vi "main.vi"() -> ()   [LabVIEW 2016]
uses:
  System Status.ctl
  Position Control.ctl
  Position Coordinate.ctl
  Manual Operation Control.ctl
panel:
  in  "Manual Operation Control":T1 {"Speed Override (%)" min=0.0 max=150.0 step=1.0 scale=0.0..150.0; "Rotative"."Step Length" min=0.01 max=100.0 step=0.01; "Rotative"."Speed" scale=0.0..500.0; "Linear"."Step Length" min=0.01 max=500.0 step=0.01; "Linear"."Speed" scale=0.0..500.0}
  in  "Settings":bool
  in  "Stop":bool
  in  "Initialize":bool
  in  "Auto Run":bool
  in  "Auto Run Control":T2[](array[typedef])
  in  "Rev Position":T3={"Pos X"=0.0, "Position Name"="Rel Move", "Pos Y"=0.0, "Pos Z"=0.0, "Pos A"=0.0, "OK Button"=FALSE, "Normal Move"=FALSE, "Fast Move"=FALSE} {"Pos A" format="%.2f"; "Pos Z" format="%.2f"; "Pos Y" format="%.2f"; "Pos X" format="%.2f"}
  in  "Abs Position":T3={"Pos X"=0.0, "Position Name"="Abs Move", "Pos Y"=0.0, "Pos Z"=0.0, "Pos A"=0.0, "OK Button"=FALSE, "Normal Move"=FALSE, "Fast Move"=FALSE} {"Pos A" format="%.2f"; "Pos Z" format="%.2f"; "Pos Y" format="%.2f"; "Pos X" format="%.2f"}
  out "System Status":T4 {"Axis A"."Position" format="%.2g"; "Axis Z"."Position" format="%.2g"; "Axis Y"."Position" format="%.2g"; "Linear Speed" format="%#.2g"; "Axis X"."Position" format="%.2g"}
  out "Error Information":string
  in  "MotionLibrary Path":path=path "C:/Program Files (x86)/National Instruments/LabVIEW 2016/user.lib/iselmotion/CNCAPI/CtrlDll/Dummy/mctlDummy.dll"
  out "Motor hModule":i32
  in  "MotionIni File In":path=path "C:/Program Files (x86)/National Instruments/LabVIEW 2016/user.lib/iselmotion/CNCAPI/CtrlDll/Dummy/MctlDummy.INI"
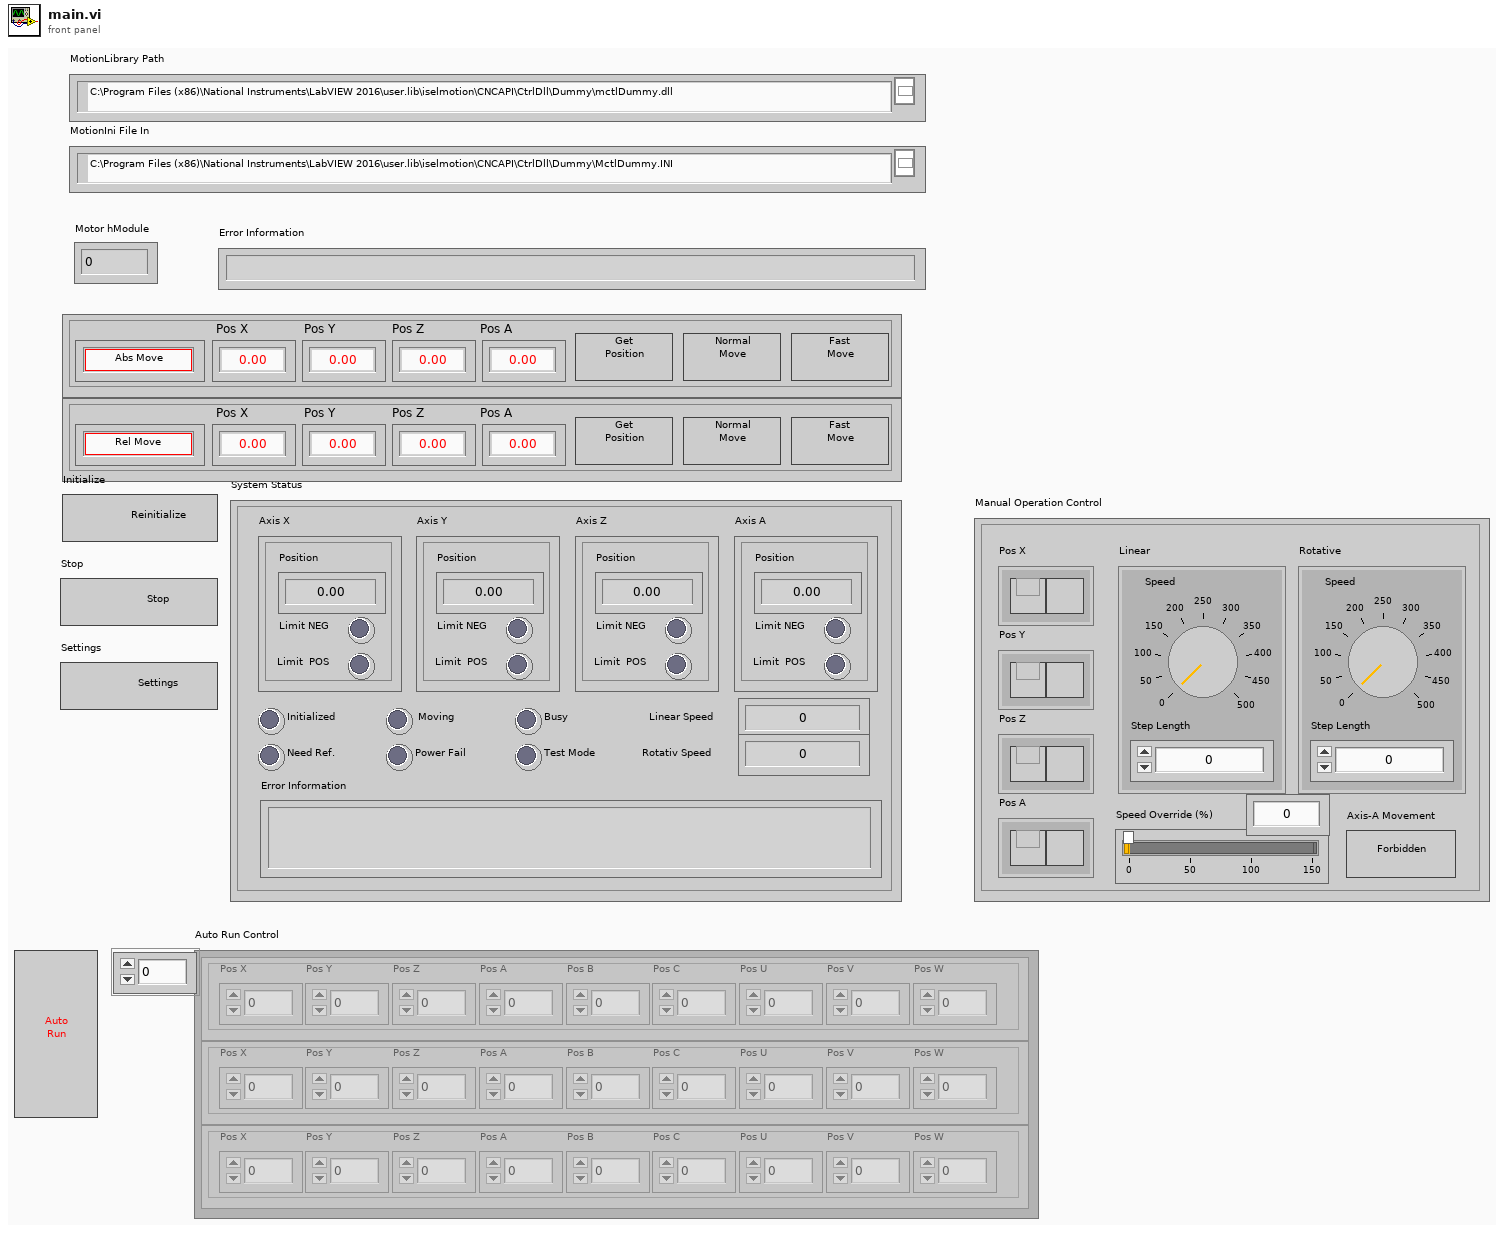
[diagram p1: front panel]
types:
  T1 = typedef "Manual Operation Control.ctl" = cluster{"Pos X":cluster{"Plus":bool, "Minus":bool}, "Pos Y":cluster{"Plus":bool, "Minus":bool}, "Pos Z":cluster{"Plus":bool, "Minus":bool}, "Pos A":cluster{"Plus":bool, "Minus":bool}, "Linear":cluster{"Speed":dbl, "Step Length":dbl}, "Rotative":cluster{"Speed":dbl, "Step Length":dbl}, "Speed Override (%)":dbl, "Axis-A Movement":bool}
  T2 = typedef "Position Coordinate.ctl" = cluster{"Pos X":dbl, "Pos Y":dbl, "Pos Z":dbl, "Pos A":dbl, "Pos B":dbl, "Pos C":dbl, "Pos U":dbl, "Pos V":dbl, "Pos W":dbl}
  T3 = typedef "Position Control.ctl" = cluster{"Pos X":dbl, "Position Name":string, "Pos Y":dbl, "Pos Z":dbl, "Pos A":dbl, "OK Button":bool, "Normal Move":bool, "Fast Move":bool}
  T4 = typedef "System Status.ctl" = cluster{"Axis X":cluster{"Position":dbl, "Limit NEG":bool, "Limit  POS":bool}, "Axis Y":cluster{"Position":dbl, "Limit NEG":bool, "Limit  POS":bool}, "Axis Z":cluster{"Position":dbl, "Limit NEG":bool, "Limit  POS":bool}, "Axis A":cluster{"Position":dbl, "Limit NEG":bool, "Limit  POS":bool}, "Initialized":bool, " Moving":bool, "Busy":bool, "Need Ref.":bool, "Power Fail":bool, "Test Mode":bool, "Linear Speed":dbl, "Rotativ Speed":dbl, "Error Information":string}
  T5 = enum16{"open", "replace", "create", "open or create", "replace or create", "replace or create with confirmation"}
  T6 = cluster{"PosX":i32, "PosY":i32, "PosZ":i32, "PosA":i32, "PosB":i32, "PosC":i32, "PosU":i32, "PosV":i32, "PosW":i32}
  T7 = cluster{"MotionLibrary Path":path, "MotionIni File In":path}
  T8 = cluster{"Common":cluster{"INMOTION":bool, "INSTOPMODE":bool, "INTEACHMODE":bool, "INTESTMODE":bool, "CURRENTOFF":bool, "INPATHMOTION":bool, "ISMOVING":bool, "PATHSTARTED":bool, "NEEDREFERENCERUN":bool, "BREAKERROR":bool, "HWLSACTIVE":bool, "SWLSACTIVE":bool, "HWLSDURINGMOTION":bool, "AFTERRUNERROR":bool, "LOADPATHDATAERROR":bool, "KEYSWITCHERROR":bool, "KEYSWDURINGMOTION":bool, "POWER_FAIL":bool, "SC_FAIL":bool, "HARDWARE_FAIL":bool, "COMMUNICATION_FAIL":bool}, "HWLSNeg":cluster{"HWLS_X_NEG":bool, "HWLS_Y_NEG":bool, "HWLS_Z_NEG":bool, "HWLS_A_NEG":bool, "HWLS_B_NEG":bool, "HWLS_C_NEG":bool, "HWLS_U_NEG":bool, "HWLS_V_NEG":bool, "HWLS_W_NEG":bool}, "HWLSPos":cluster{"HWLS_X_POS":bool, "HWLS_Y_POS":bool, "HWLS_Z_POS":bool, "HWLS_A_POS":bool, "HWLS_B_POS":bool, "HWLS_C_POS":bool, "HWLS_U_POS":bool, "HWLS_V_POS":bool, "HWLS_W_POS":bool}, "SWLSNeg":cluster{"SWLS_X_NEG":bool, "SWLS_Y_NEG":bool, "SWLS_Z_NEG":bool, "SWLS_A_NEG":bool, "SWLS_B_NEG":bool, "SWLS_C_NEG":bool, "SWLS_U_NEG":bool, "SWLS_V_NEG":bool, "SWLS_W_NEG":bool}, "SWLSPos":cluster{"SWLS_X_POS":bool, "SWLS_Y_POS":bool, "SWLS_Z_POS":bool, "SWLS_A_POS":bool, "SWLS_B_POS":bool, "SWLS_C_POS":bool, "SWLS_U_POS":bool, "SWLS_V_POS":bool, "SWLS_W_POS":bool}, "Extended":cluster{"ISBUSY":bool, "DISABLED":bool, "ISINITIALIZED":bool, "READY":bool, "DRILLCYCLEACTIVE":bool, "CTRLSPECERROR":bool}, "Additional flags":cluster{"InMotion":bool, "InStopMode":bool, "InTeachMode":bool, "InTestMode":bool, "CurrentOff":bool, "InPathMotion":bool, "IsMoving":bool, "NeedReferenceRun":bool, "BreakError":bool, "HWLSActive":bool, "SWLSActive":bool, "HWLSDuringMotion":bool, "AfterRunError":bool, "PowerFail":bool, "SCFail":bool, "IsBusy":bool, "Initialized":bool, "Disabled":bool, "HardwareFail":bool, "CommunicationFail":bool, "DrillCycleActive":bool, "CtrlSpecError":bool, "PathStarted":bool}}
  T9 = cluster{"PosX":dbl, "PosY":dbl, "PosZ":dbl, "PosA":dbl, "PosB":dbl, "PosC":dbl, "PosU":dbl, "PosV":dbl, "PosW":dbl}
  T10 = cluster{"PosX":dbl, "HWLS_X_NEG":bool, "HWLS_X_POS":bool}
  T11 = cluster{"PosY":dbl, "HWLS_Y_NEG":bool, "HWLS_Y_POS":bool}
  T12 = cluster{"PosZ":dbl, "HWLS_Z_NEG":bool, "HWLS_Z_POS":bool}
  T13 = cluster{dbl, "HWLS_A_NEG":bool, "HWLS_A_POS":bool}
  T14 = cluster{"LiNormVel":i32, "DrNormVel":i32, "LiFastVel":i32, "DrFastVel":i32, "LiTeachVel":i32, "DrTeachVel":i32, "LiActVel":i32, "DrActVel":i32}
  T15 = cluster{"LiNormVel":dbl, "DrNormVel":dbl, "LiFastVel":dbl, "DrFastVel":dbl, "LiTeachVel":dbl, "DrTeachVel":dbl, "LiActVel":dbl, "DrActVel":dbl}
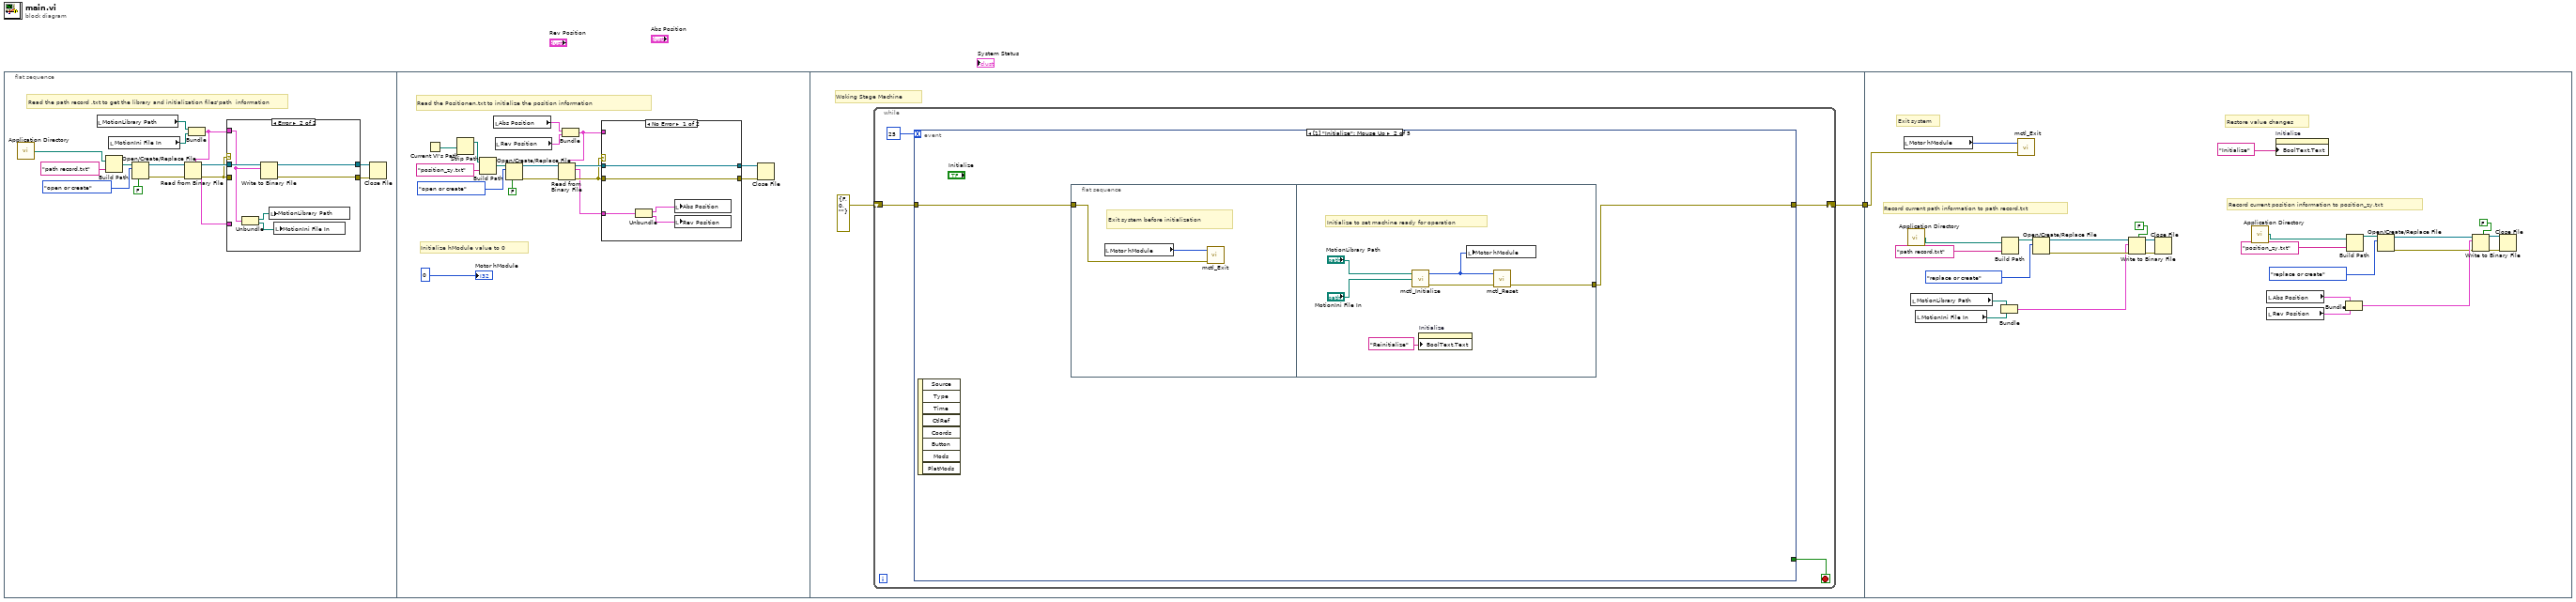
[diagram p0: block diagram]
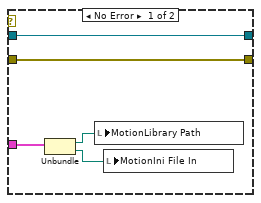
[diagram p2: hidden frame]
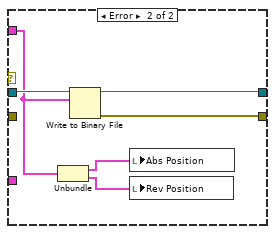
[diagram p3: hidden frame]
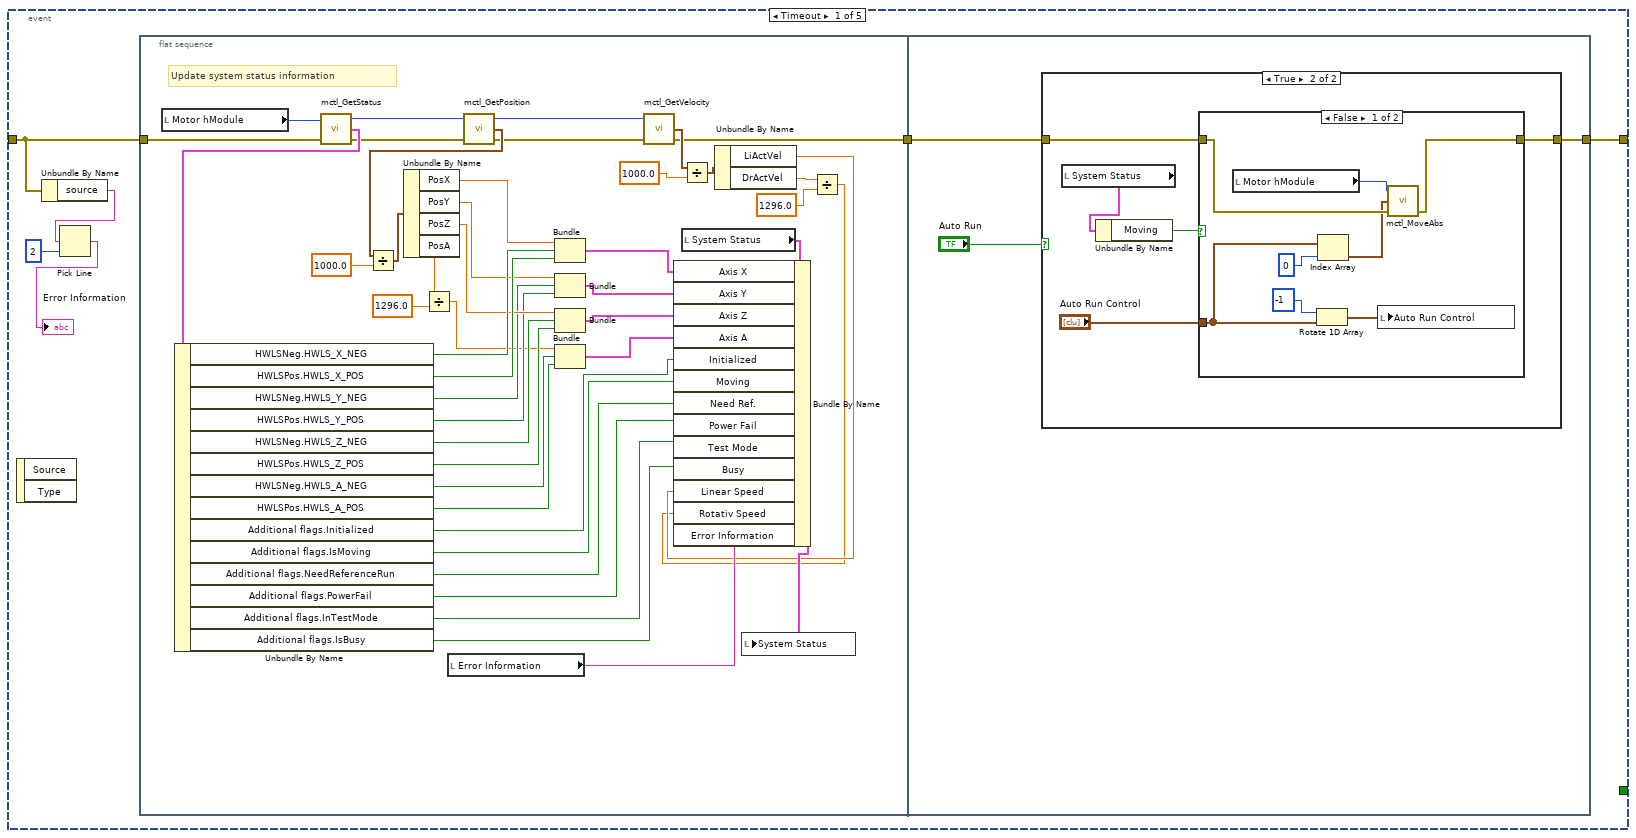
[diagram p4: hidden frame]
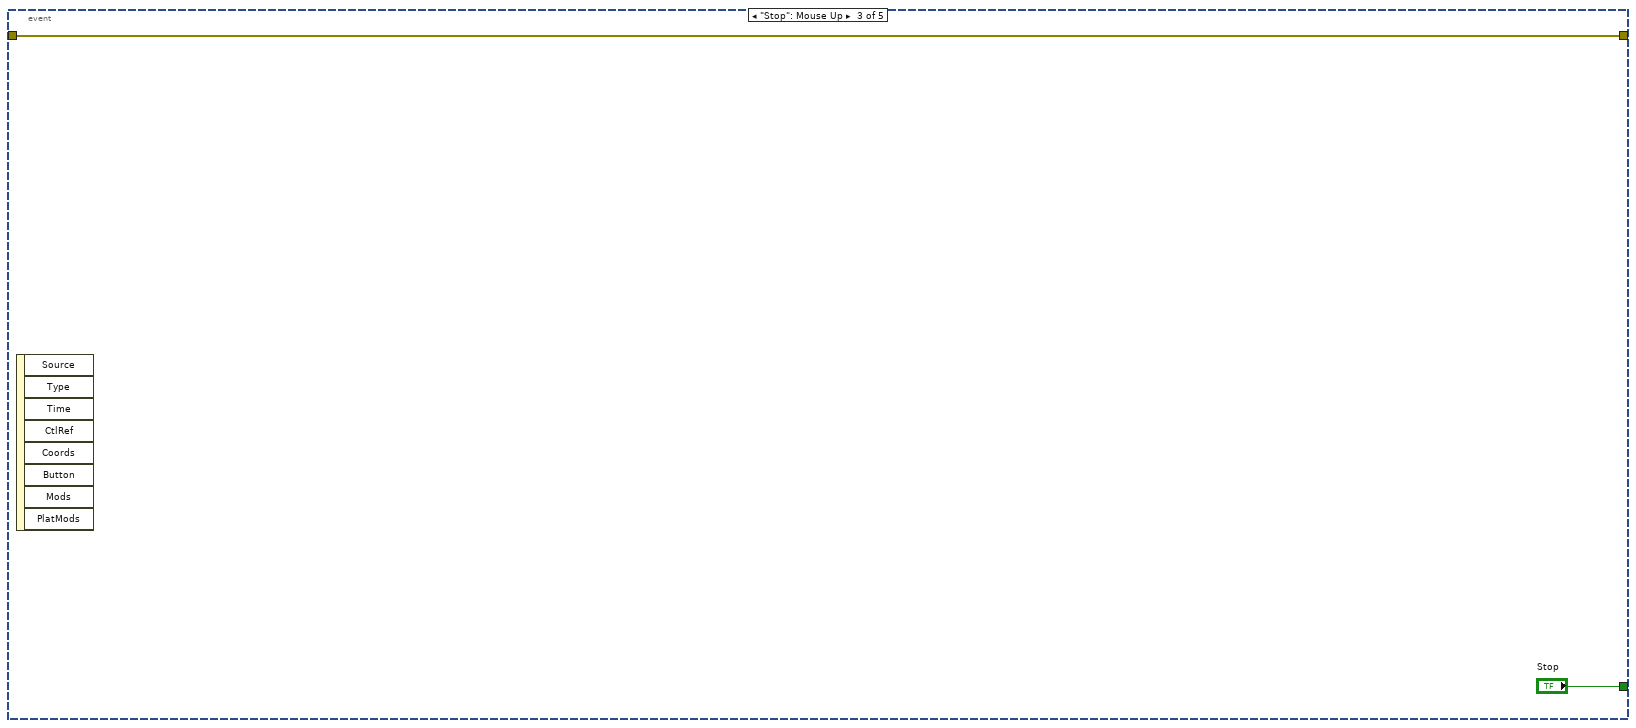
[diagram p7: hidden frame]
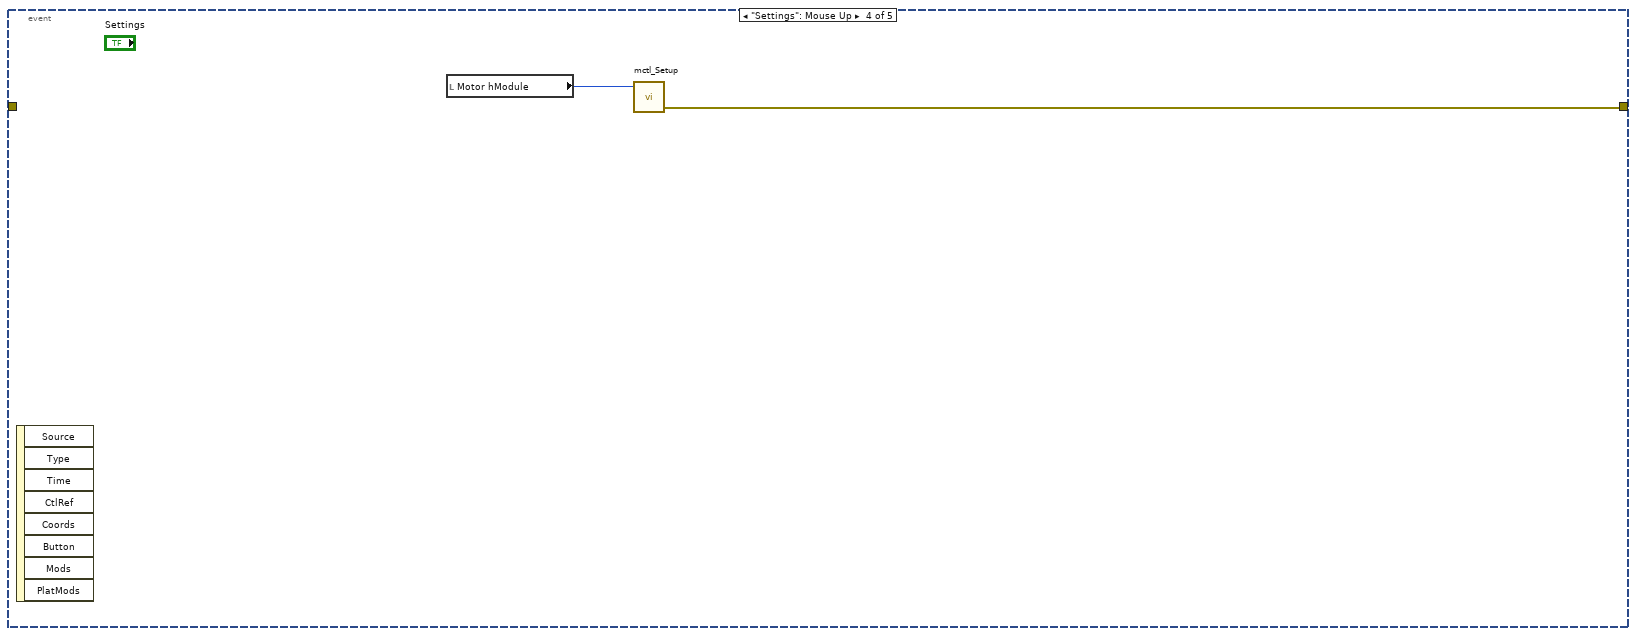
[diagram p8: hidden frame]
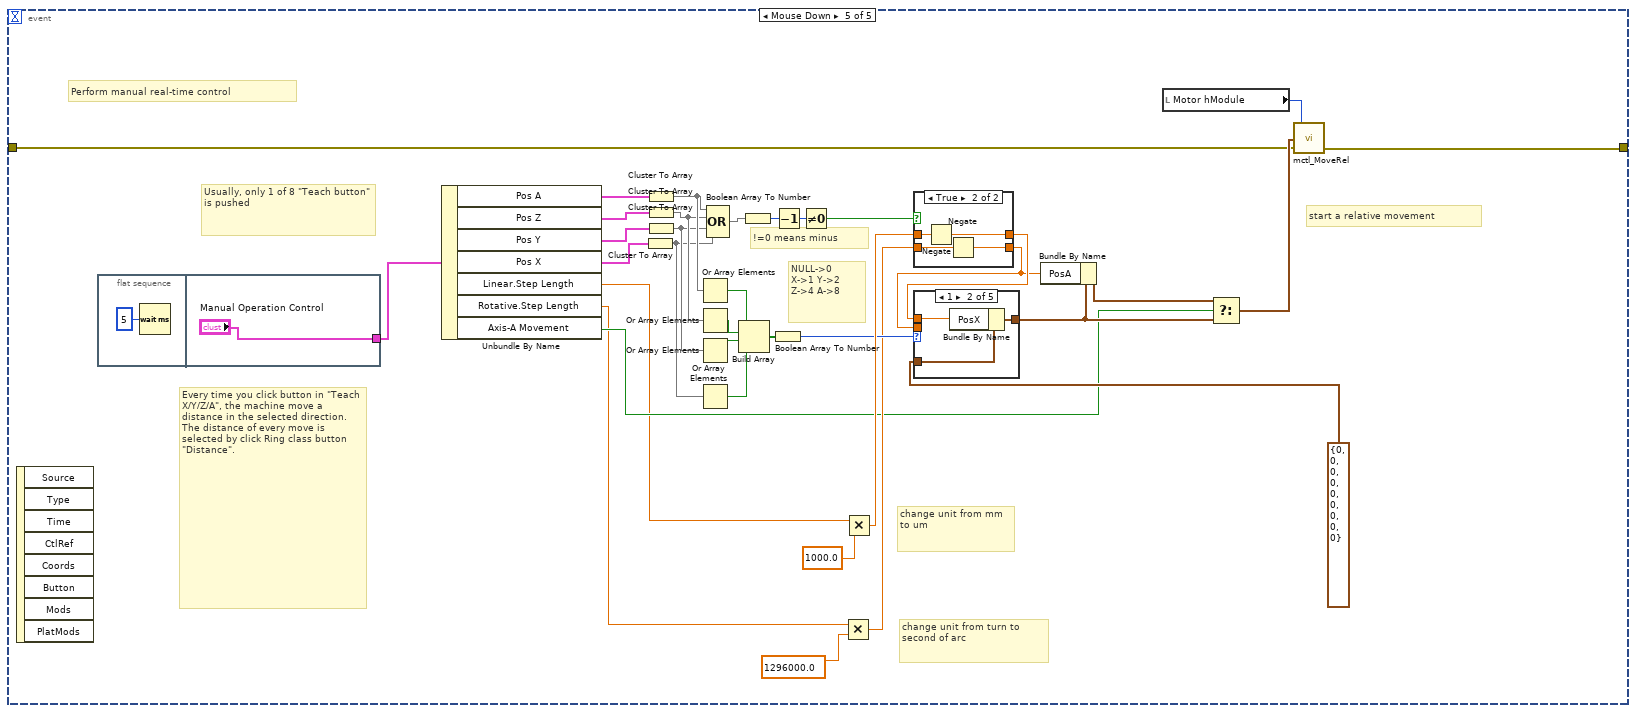
[diagram p9: hidden frame]
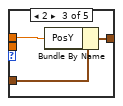
[diagram p11: hidden frame]
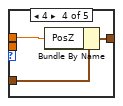
[diagram p12: hidden frame]
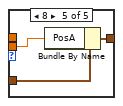
[diagram p13: hidden frame]
diagram:
  n1 = flat-sequence {
    tunnel: [w56] -> w1
    tunnel: w1 -> [w201]
    frame #0 {
      # "Read the path record .txt to get the library and initialization files'path  information"
      n2 = call <vilib>:"Application Directory.vi"() -> ("Application Directory"=w3:path)
      n3 = local read "MotionLibrary Path"() -> (w11:path)
      n4 = Build Path(base path=w3, name or relative path="path record.txt") -> (appended path=w14:path)
      n5 = local read "MotionIni File In"() -> (w12:path)
      n6 = Open/Create/Replace File(file path (use dialog)=w14, operation (0:open)=T5."open or create", disable buffering (F)=FALSE ("advisory dialog? (display:T)")) -> (refnum out=w16:refnum<file>, error out=w13:errorcluster)  [unwired: 3 in, 1 out]
      n7 = Bundle("MotionLibrary Path"=w11, "MotionIni File In"=w12) -> (w4:T7)  [unwired: 1 in]
      n8 = Read from Binary File(5:w4, 8:w13, 11:w16) -> (0:w5:errorcluster, 2:w2:T7, 3:w8:refnum<file>)  [unwired: 3 in, 1 out]
      n9 = case shown="Error" w5 {
        tunnel: w8 -> [w21 w27]
        tunnel: [w21 w25] -> w7
        tunnel: [w20 w26] -> w6
        tunnel: w5 -> [w20 _]
        tunnel: w4 -> [_ w24]
        tunnel: w2 -> [w19 _]
        frame No Error {
          n10 = Unbundle(w19) -> ("MotionLibrary Path"=w18:path, "MotionIni File In"=w17:path)
          n11 = local write "MotionLibrary Path"(w18) -> ()
          n12 = local write "MotionIni File In"(w17) -> ()
        }
        frame Error {
          n13 = Unbundle(w24) -> ("MotionLibrary Path"=w23:path, "MotionIni File In"=w22:path)
          n14 = Write to Binary File(file (use dialog)=w27, data=w24) -> (refnum out=w25:refnum<file>, error out=w26:errorcluster)  [unwired: 4 in, 1 out]
          n15 = local write "MotionLibrary Path"(w23) -> ()
          n16 = local write "MotionIni File In"(w22) -> ()
        }
      }
      n17 = Close File(refnum=w7, error in=w6) -> ()  [unwired: 2 out]
    }
    frame #1 {
      # "Initialize hModule value to 0"
      # "Read the Positionen.txt to initialize the position information"
      n18 = Current VI's Path() -> (path=w30:path)
      n19 = Strip Path(path=w30) -> (stripped path=w43:path)  [unwired: 1 out]
      n20 = Build Path(base path=w43, name or relative path="position_zy.txt") -> (appended path=w41:path)
      n21 = local read "Abs Position"() -> (w38:T3)
      n22 = local read "Rev Position"() -> (w39:T3)
      n23 = Open/Create/Replace File(file path (use dialog)=w41, operation (0:open)=T5."open or create", disable buffering (F)=FALSE ("advisory dialog? (display:T)")) -> (refnum out=w44:refnum<file>, error out=w40:errorcluster)  [unwired: 3 in, 1 out]
      n24 = Bundle("Abs Position"=w38, "Rev Position"=w39) -> (w31:cluster{"Abs Position":T3, "Rev Position":T3})  [unwired: 1 in]
      n25 = Read from Binary File(5:w31, 8:w40, 11:w44) -> (0:w32:errorcluster, 2:w28:cluster{"Abs Position":T3, "Rev Position":T3}, 3:w35:refnum<file>)  [unwired: 3 in, 1 out]
      n26 = case shown="No Error" w32 {
        tunnel: w35 -> [w49 w55]
        tunnel: [w49 w53] -> w34
        tunnel: [w48 w54] -> w33
        tunnel: w32 -> [w48 _]
        tunnel: w31 -> [_ w52]
        tunnel: w28 -> [w47 _]
        frame No Error {
          n27 = Unbundle(w47) -> ("Abs Position"=w46:T3, "Rev Position"=w45:T3)
          n28 = local write "Abs Position"(w46) -> ()
          n29 = local write "Rev Position"(w45) -> ()
        }
        frame Error {
          n30 = Unbundle(w52) -> ("Abs Position"=w51:T3, "Rev Position"=w50:T3)
          n31 = Write to Binary File(file (use dialog)=w55, data=w52) -> (refnum out=w53:refnum<file>, error out=w54:errorcluster)  [unwired: 4 in, 1 out]
          n32 = local write "Abs Position"(w51) -> ()
          n33 = local write "Rev Position"(w50) -> ()
        }
      }
      n34 = Close File(refnum=w34, error in=w33) -> ()  [unwired: 2 out]
      "Motor hModule" <- 0
    }
    frame #2 {
      # "Woking Stage Machine"
      n35 = while {
        shift-right: [w59] -> w56
        shift-left: errorcluster {"status"=FALSE, "code"=0, "source"=""} ("error constant") -> [w60]
        stop <- w58 stop-if-true
        n36 = event shown="[1] \"Initialize\": Mouse Up" {
          selector: _ -> [_ _ _ _ _]
          dyn-events: _ -> [_ _ _ _ _]
          timeout: 25 -> [_ _ _ _ _]
          tunnel: w60 -> [w67 w131 w141 _ w149]
          tunnel: [w62 w132 w141 w143 w147] -> w59
          tunnel: [_ _ "Stop" _ _] -> w58
          event Timeout {
            n37 = event-data() -> ()  [unwired: 1 in, 2 out]
            n38 = Unbundle By Name(w67) -> ("source"=w65:string)
            n39 = Pick Line(multi-line string=w65, line index=2) -> (output string=→"Error Information":string)  [unwired: 1 in]
            n40 = flat-sequence {
              tunnel: w67 -> [w71]
              tunnel: [w68] -> w63
              tunnel: w63 -> [w114]
              tunnel: [w113] -> w62
              frame #0 {
                # "Update system status information"
                n41 = local read "Motor hModule"() -> (w112:i32)
                n42 = call <userlib>:"mctl_GetStatus.vi"("error in"=w71, "hModule In"=w112) -> ("error out"=w70:errorcluster, "Status"=w111:T8, "hModule Out"=w110:u32)  [unwired: 1 in]
                n43 = Unbundle By Name(w111) -> ("HWLSNeg.HWLS_X_NEG"=w104:bool, "HWLSPos.HWLS_X_POS"=w103:bool, "HWLSNeg.HWLS_Y_NEG"=w100:bool, "HWLSPos.HWLS_Y_POS"=w99:bool, "HWLSNeg.HWLS_Z_NEG"=w98:bool, "HWLSPos.HWLS_Z_POS"=w97:bool, "HWLSNeg.HWLS_A_NEG"=w96:bool, "HWLSPos.HWLS_A_POS"=w95:bool, "Additional flags.Initialized"=w90:bool, "Additional flags.IsMoving"=w89:bool, "Additional flags.NeedReferenceRun"=w88:bool, "Additional flags.PowerFail"=w85:bool, "Additional flags.InTestMode"=w86:bool, "Additional flags.IsBusy"=w87:bool)
                n44 = local read "Error Information"() -> (w84:string)
                n45 = call <userlib>:"mctl_GetPosition.vi"("error in"=w70, "hModule In"=w110) -> ("error out"=w69:errorcluster, "AxisPos"=w108:T6, "hModule Out"=w109:u32)  [unwired: 1 in]
                n46 = Divide(x=w108, y=1000.0) -> (x/y=w106:T9)
                n47 = Unbundle By Name(w106) -> ("PosX"=w105:dbl, "PosY"=w102:dbl, "PosZ"=w101:dbl, "PosA"=w81:dbl)
                n48 = Divide(x=w81, y=1296.0) -> (x/y=w79:dbl)
                n49 = Bundle("PosX"=w105, "HWLS_X_NEG"=w104, "HWLS_X_POS"=w103) -> (w94:T10)  [unwired: 1 in]
                n50 = Bundle("PosY"=w102, "HWLS_Y_NEG"=w100, "HWLS_Y_POS"=w99) -> (w93:T11)  [unwired: 1 in]
                n51 = Bundle("PosZ"=w101, "HWLS_Z_NEG"=w98, "HWLS_Z_POS"=w97) -> (w92:T12)  [unwired: 1 in]
                n52 = Bundle(w79, "HWLS_A_NEG"=w96, "HWLS_A_POS"=w95) -> (w91:T13)  [unwired: 1 in]
                n53 = call <userlib>:"mctl_GetVelocity.vi"("error in"=w69, "hModule In"=w109) -> ("error out"=w68:errorcluster, "Velocity"=w76:T14)  [unwired: 1 in, 1 out]
                n54 = Divide(x=w76, y=1000.0) -> (x/y=w77:T15)
                n55 = local read "System Status"() -> (w83:T4)
                n56 = Unbundle By Name(w77) -> ("LiActVel"=w78:dbl, "DrActVel"=w74:dbl)
                n57 = Divide(x=w74, y=1296.0) -> (x/y=w72:dbl)
                n58 = Bundle By Name(cluster=w83, "Axis X"=w94, "Axis Y"=w93, "Axis Z"=w92, "Axis A"=w91, "Initialized"=w90, "Moving"=w89, "Need Ref."=w88, "Power Fail"=w85, "Test Mode"=w86, "Busy"=w87, "Linear Speed"=w78, "Rotativ Speed"=w72, "Error Information"=w84) -> (w82:T4)
                n59 = local write "System Status"(w82) -> ()
              }
              frame #1 {
                n60 = case shown="True" "Auto Run" {
                  tunnel: w114 -> [w116 w119]
                  tunnel: [w116 w118] -> w113
                  frame False {
                  }
                  frame True {
                    n61 = local read "System Status"() -> (w120:T4)
                    n62 = Unbundle By Name(w120) -> ("Moving"=w121:bool)
                    n63 = case shown="False" w121 {
                      tunnel: w119 -> [w127 w130]
                      tunnel: [w123 w130] -> w118
                      tunnel: "Auto Run Control" -> [w125 _]
                      frame False {
                        n64 = local read "Motor hModule"() -> (w126:i32)
                        n65 = Rotate 1D Array(1:w125, 2:-1 ("n")) -> (0:w122:T2[])
                        n66 = Index Array(array=w125, index=0) -> (element=w124:T2)
                        n67 = local write "Auto Run Control"(w122) -> ()
                        n68 = call <userlib>:"mctl_MoveAbs.vi"("error in"=w127, "Abs"=w124, "hModule In"=w126) -> ("error out"=w123:errorcluster)  [unwired: 1 in, 1 out]
                      }
                      frame True {
                      }
                    }
                  }
                }
              }
            }
          }
          event "Initialize": Mouse Up {
            n69 = event-data() -> ()  [unwired: 1 in, 8 out]
            n70 = flat-sequence {
              tunnel: w131 -> [w133]
              tunnel: [w139] -> w132
              frame #0 {
                # "Exit system before initialization"
                n71 = local read "Motor hModule"() -> (w134:i32)
                n72 = call <userlib>:"mctl_Exit.vi"("error in"=w133, "hModule In"=w134) -> ()  [unwired: 2 in, 2 out]
              }
              frame #1 {
                # "Initialize to set machine ready for operation"
                n73 = call <userlib>:"mctl_Initialize.vi"("Ini File In"="MotionIni File In", "Library In"="MotionLibrary Path") -> ("error out"=w140:errorcluster, "hModule Out"=w136:u32)  [unwired: 1 in, 1 out]
                n74 = property on="Initialize" class="Bool (strict)"("BoolText.Text"="Reinitialize" ("Boolean Text.Text")) -> ()  [unwired: 2 in, 2 out]
                n75 = local write "Motor hModule"(w136) -> ()
                n76 = call <userlib>:"mctl_Reset.vi"("error in"=w140, "hModule In"=w136) -> ("error out"=w139:errorcluster)  [unwired: 2 in, 1 out]
              }
            }
          }
          event "Stop": Mouse Up {
            n77 = event-data() -> ()  [unwired: 1 in, 8 out]
          }
          event "Settings": Mouse Up {
            n78 = event-data() -> ()  [unwired: 1 in, 8 out]
            n79 = local read "Motor hModule"() -> (w144:i32)
            n80 = call <userlib>:"mctl_Setup.vi"("hModule In"=w144) -> ("error out"=w143:errorcluster)  [unwired: 3 in, 1 out]
          }
          event Mouse Down {
            # "Usually, only 1 of 8 \"Teach button\" is pushed"
            # "!=0 means minus"
            # "change unit from turn to second of arc"
            # "change unit from mm to um"
            # "start a relative movement"
            # "Every time you click button in \"Teach X/Y/Z/A\", the machine move a distance in the selected direction. The distance of every move is selected by click Ring class button \"Distance\"."
            # "NULL->0\nX->1 Y->2\nZ->4 A->8"
            # "Perform manual real-time control"
            n81 = event-data() -> ()  [unwired: 1 in, 8 out]
            n82 = flat-sequence {
              tunnel: ["Manual Operation Control"] -> w151
              frame #0 {
                n83 = Wait (ms)(milliseconds to wait=u32 5) -> ()  [unwired: 1 out]
              }
              frame #1 {
              }
            }
            n84 = Unbundle By Name(w151) -> ("Pos A"=w179:cluster{"Plus":bool, "Minus":bool}, "Pos Z"=w178:cluster{"Plus":bool, "Minus":bool}, "Pos Y"=w177:cluster{"Plus":bool, "Minus":bool}, "Pos X"=w176:cluster{"Plus":bool, "Minus":bool}, "Linear.Step Length"=w146:dbl, "Rotative.Step Length"=w145:dbl, "Axis-A Movement"=w152:bool)
            n85 = Cluster To Array(cluster=w176) -> (array=w167:bool[])
            n86 = Cluster To Array(cluster=w179) -> (array=w170:bool[])
            n87 = Cluster To Array(cluster=w178) -> (array=w169:bool[])
            n88 = Cluster To Array(cluster=w177) -> (array=w168:bool[])
            n89 = Or Array Elements(Boolean array=w170) -> (logical OR=w175:bool)
            n90 = Or Array Elements(Boolean array=w169) -> (logical OR=w174:bool)
            n91 = Or Array Elements(Boolean array=w168) -> (logical OR=w173:bool)
            n92 = Or Array Elements(Boolean array=w167) -> (logical OR=w172:bool)
            n93 = Compound Arithmetic op=OR(w170, w169, w168, w167) -> (w164:bool[])
            n94 = Build Array(w175, w174, w173, w172) -> (w171:bool[])
            n95 = Boolean Array To Number(Boolean array=w164) -> (number=w166:u32)
            n96 = Boolean Array To Number(Boolean array=w171) -> (number=w161:u32)
            n97 = Decrement(x=w166) -> (x-1=w165:u32)
            n98 = Not Equal To 0?(x=w165) -> (x != 0?=w150:bool)
            n99 = Multiply(x=w145, y=1296000.0) -> (x*y=w157:dbl)
            n100 = Multiply(x=w146, y=1000.0) -> (x*y=w162:dbl)
            n101 = case shown="True" w150 {
              tunnel: w162 -> [w196 w200]
              tunnel: [w196 w199] -> w159
              tunnel: w157 -> [w195 w198]
              tunnel: [w195 w197] -> w155
              frame False {
              }
              frame True {
                n102 = Negate(x=w200) -> (-x=w199:dbl)
                n103 = Negate(x=w198) -> (-x=w197:dbl)
              }
            }
            n104 = case shown="1" w161 {
              tunnel: T6 {"PosX"=0, "PosY"=0, "PosZ"=0, "PosA"=0, "PosB"=0, "PosC"=0, "PosU"=0, "PosV"=0, "PosW"=0} ("RelPOS") -> [w182 w184 w187 w190 w193]
              tunnel: [w182 w185 w188 w191 w194] -> w156
              tunnel: w159 -> [_ w183 w186 w189 _]
              tunnel: w155 -> [_ _ _ _ w192]
              frame 0, Default {
              }
              frame 1 {
                n105 = Bundle By Name(cluster=w184, "PosX"=w183) -> (w185:T6)
              }
              frame 2 {
                n106 = Bundle By Name(cluster=w187, "PosY"=w186) -> (w188:T6)
              }
              frame 4 {
                n107 = Bundle By Name(cluster=w190, "PosZ"=w189) -> (w191:T6)
              }
              frame 8 {
                n108 = Bundle By Name(cluster=w193, "PosA"=w192) -> (w194:T6)
              }
            }
            n109 = Bundle By Name(cluster=w156, "PosA"=w155) -> (w154:T6)
            n110 = local read "Motor hModule"() -> (w148:i32)
            n111 = Select(t=w154, s=w152, f=w156) -> (s? t:f=w153:T6)
            n112 = call <userlib>:"mctl_MoveRel.vi"("error in"=w149, "RelPOS"=w153, "hModule In"=w148) -> ("error out"=w147:errorcluster)  [unwired: 1 in, 1 out]
          }
        }
      }
    }
    frame #3 {
      # "Exit system"
      # "Restore value changes"
      # "Record current position information to position_zy.txt"
      # "Record current path information to path record.txt"
      n113 = local read "Motor hModule"() -> (w202:i32)
      n114 = call <vilib>:"Application Directory.vi"() -> ("Application Directory"=w217:path)
      n115 = local read "MotionLibrary Path"() -> (w221:path)
      n116 = local read "MotionIni File In"() -> (w220:path)
      n117 = Bundle("MotionLibrary Path"=w221, "MotionIni File In"=w220) -> (w219:T7)  [unwired: 1 in]
      n118 = Build Path(base path=w217, name or relative path="path record.txt") -> (appended path=w226:path)
      n119 = call <userlib>:"mctl_Exit.vi"("error in"=w201, "hModule In"=w202) -> ()  [unwired: 2 in, 2 out]
      n120 = Open/Create/Replace File(file path (use dialog)=w226, operation (0:open)=T5."replace or create") -> (refnum out=w225:refnum<file>, error out=w223:errorcluster)  [unwired: 4 in, 1 out]
      n121 = Write to Binary File(file (use dialog)=w225, data=w219, error in=w223, 5:FALSE ("prepend array or string size? (T)")) -> (refnum out=w224:refnum<file>, error out=w222:errorcluster)  [unwired: 2 in, 1 out]
      n122 = Close File(refnum=w224, error in=w222) -> ()  [unwired: 2 out]
      n123 = call <vilib>:"Application Directory.vi"() -> ("Application Directory"=w214:path)
      n124 = local read "Abs Position"() -> (w210:T3)
      n125 = local read "Rev Position"() -> (w211:T3)
      n126 = property on="Initialize" class="Bool (strict)"("BoolText.Text"="Initialize" ("Boolean Text.Text")) -> ()  [unwired: 2 in, 2 out]
      n127 = Bundle("Abs Position"=w210, "Rev Position"=w211) -> (w212:cluster{"Abs Position":T3, "Rev Position":T3})  [unwired: 1 in]
      n128 = Build Path(base path=w214, name or relative path="position_zy.txt") -> (appended path=w205:path)
      n129 = Open/Create/Replace File(file path (use dialog)=w205, operation (0:open)=T5."replace or create") -> (refnum out=w206:refnum<file>, error out=w208:errorcluster)  [unwired: 4 in, 1 out]
      n130 = Write to Binary File(file (use dialog)=w206, data=w212, error in=w208, 5:FALSE ("prepend array or string size? (T)")) -> (refnum out=w207:refnum<file>, error out=w209:errorcluster)  [unwired: 2 in, 1 out]
      n131 = Close File(refnum=w207, error in=w209) -> ()  [unwired: 2 out]
    }
  }
